vi "读取数据.vi"(6 "簇":T1={"VISA resource name"="", "baud rate (9600)"=9600, "data bits (8)"=8, "parity (0:none)"=enum."None", "stop bits (10: 1 bit)"=10, "timeout (10sec)"=10000} {"stop bits (10: 1 bit)" items=["1.0"=10, "1.5"=15, "2.0"=20]}) -> (1 "读取数据":u32[](array[numeric]))   [LabVIEW 2012]
panel:
  out "主PLC通讯等待延时":dbl
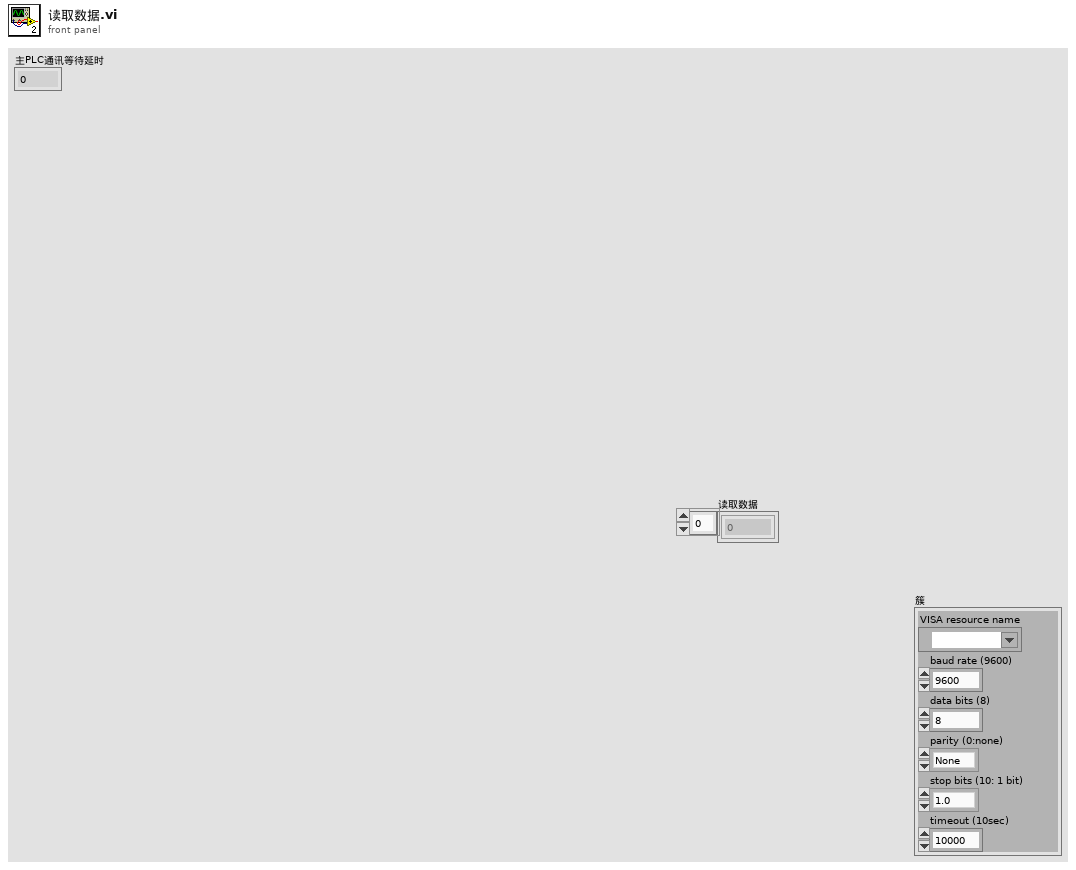
[diagram p1: front panel]
types:
  T1 = cluster{"VISA resource name":refnum<visa-resource-name>, "baud rate (9600)":u32, "data bits (8)":u16, "parity (0:none)":enum16{"None", "Odd", "Even", "Mark", "Space"}, "stop bits (10: 1 bit)":u16, "timeout (10sec)":u32}
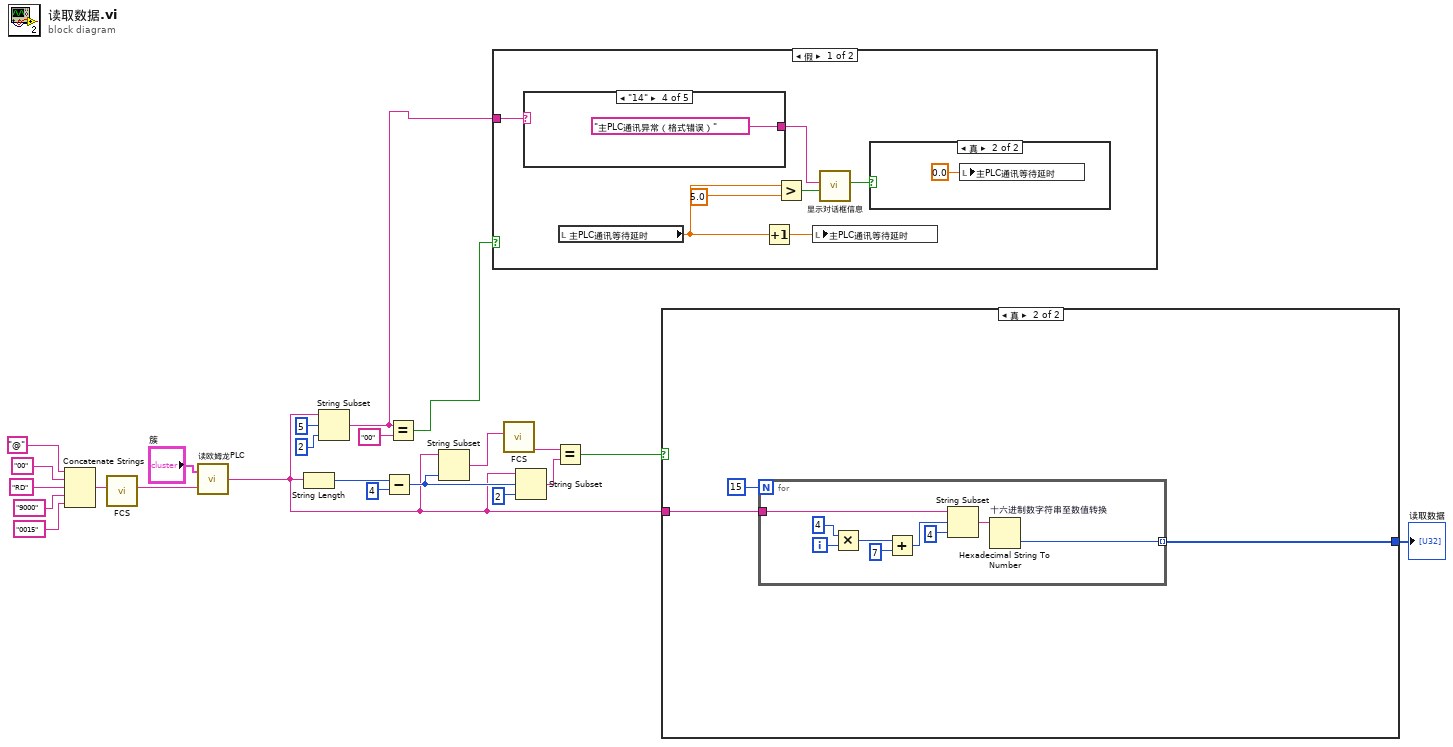
[diagram p0: block diagram]
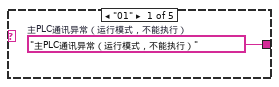
[diagram p3: hidden frame]
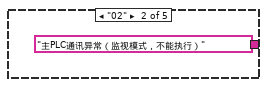
[diagram p4: hidden frame]
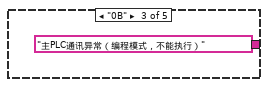
[diagram p5: hidden frame]
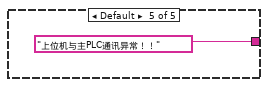
[diagram p6: hidden frame]
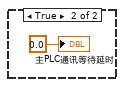
[diagram p8: hidden frame]
diagram:
  n1 = Concatenate Strings("@" ("字符串"), "00" ("字符串"), "RD" ("字符串"), "9000" ("字符串"), "0015" ("字符串")) -> (w9:string)
  n2 = call "FCS.vi"("发送命令"=w9) -> ("完整帧"=w7:string)  [unwired: 9 in, 1 out]
  n3 = call "读欧姆龙PLC.vi"("写入缓冲区"=w7, "簇"="簇") -> ("读取缓冲区"=w8:string)
  n4 = String Length(string=w8) -> (length=w11:i32)
  n5 = String Subset(string=w8, offset (0)=5 ("偏移量(0)"), length (rest)=2 ("长度（剩余）")) -> (substring=w1:string)
  n6 = Subtract(x=w11, y=4) -> (x-y=w13:i32)
  n7 = Equal?(x=w1, y="00") -> (x = y?=w10:bool)
  n8 = String Subset(string=w8, length (rest)=w13) -> (substring=w5:string)  [unwired: 1 in]
  n9 = case shown="假" w10 {
    tunnel: w1 -> [w25 _]
    frame False {
      n10 = case shown="\"14\"" w25 {
        tunnel: [w31 "主PLC通讯异常（监视模式，不能执行）" "主PLC通讯异常（编程模式，不能执行）" "主PLC通讯异常（格式错误）" "上位机与主PLC通讯异常！！"] -> w24
        frame "01" {
          w31 = "主PLC通讯异常（运行模式，不能执行）"  # 主PLC通讯异常（运行模式，不能执行）
        }
        frame "02" {
        }
        frame "0B" {
        }
        frame "14" {
        }
        frame Default {
        }
      }
      n11 = local read "主PLC通讯等待延时"() -> (w27:dbl)
      n12 = Increment(x=w27) -> (x+1=w28:dbl)
      n13 = Greater?(x=w27, y=5.0) -> (0:w29:bool)
      n14 = local write "主PLC通讯等待延时"(w28) -> ()
      n15 = call "显示对话框信息"("Enable"=w29, "Message"=w24) -> ("确定"=w26:bool)  [unwired: 8 in, 1 out]
      n16 = case shown="真" w26 {
        frame False {
        }
        frame True {
          n17 = local write "主PLC通讯等待延时"(0.0 ("主PLC通讯等待延时")) -> ()
        }
      }
    }
    frame True {
      "主PLC通讯等待延时" <- 0.0 ("数值")
    }
  }
  n18 = call "FCS.vi"("发送命令"=w5) -> ("FCS校验"=w4:string)  [unwired: 9 in, 1 out]
  n19 = String Subset(string=w8, offset (0)=w13, length (rest)=2 ("长度（剩余）")) -> (substring=w15:string)
  n20 = Equal?(x=w4, y=w15) -> (x = y?=w3:bool)
  n21 = case shown="真" w3 {
    tunnel: w8 -> [_ w39]
    tunnel: [_ w38] -> w2
    frame False {
    }
    frame True {
      n22 = for {
        N: 15 -> [_]
        tunnel: [w42] -> w38 mode=indexing
        tunnel: w39 -> [w41]
        i -> [w48]
        n23 = Multiply(x=4, y=w48) -> (x*y=w46:i32)
        n24 = Add(x=w46, y=7) -> (x+y=w44:i32)
        n25 = String Subset(string=w41, offset (0)=w44, length (rest)=4 ("长度（剩余）")) -> (substring=w49:string)
        n26 = Hexadecimal String To Number "十六进制数字符串至数值转换"(string=w49) -> (number=w42:u32)  [unwired: 2 in, 1 out]
      }
    }
  }
  "读取数据" <- w2
